vi "servo analog pin.vi"() -> ()   [LabVIEW 2022 SP3]
panel:
  in  "Amplitude":dbl=2.5
  in  "Offset":dbl=2.5
  in  "Frequency":dbl=50.0
  out "Square":dynamicdata(graph)
  in  "stop (F)":bool
  in  "Duty Cycle (%)":dbl(slide)=50.0 scale=0.0..150.0
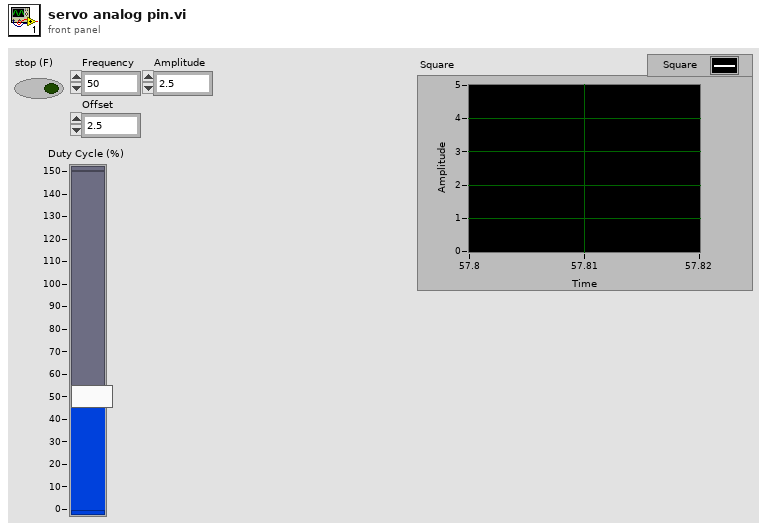
[diagram p1: front panel]
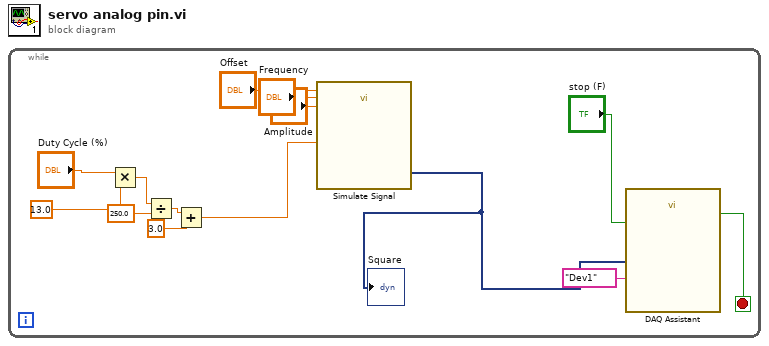
[diagram p0: block diagram]
diagram:
  n1 = while {
    stop <- w13 stop-if-true
    n2 = Multiply(x="Duty Cycle (%)", y=13.0) -> (x*y=w7:dbl)
    n3 = Divide(x=w7, y=250.0) -> (x/y=w6:dbl)
    n4 = Add(x=w6, y=3.0) -> (x+y=w1:dbl)
    n5 = call "Simulate Signal"("Offset"="Offset", "Duty Cycle (%)"=w1, "Frequency"="Frequency", "Amplitude"="Amplitude") -> ("Square"=w9:dynamicdata)  [unwired: 10 in, 1 out]
    "Square" <- w9
    n6 = call "DAQ Assistant"("data"=w9, "stop (F)"="stop (F)", "device name"=tag "Dev1") -> ("stopped"=w13:bool)  [unwired: 14 in, 2 out]
  }
